vi "TestExampleCD.vi"() -> ()   [LabVIEW 2012]
uses:
  ExampleClassC/ExampleClassC.lvclass
  ExampleClassDEdge/ExampleClassDEdge.lvclass
  ExampleClassDInverse/ExampleClassDInverse.lvclass
  ExampleClassDMath/ExampleClassDKaleidoscope/ExampleClassDMath.lvclass
  ExampleClassDScaffold/ExampleClassDScaffold.lvclass
  <vilib>/Distrio/Murmex/Murmex/Murmex.lvclass
panel:
  in  "method":enum16{"Inverse", "Edge", "Math"}(ring)
  # "Test Example C & D"
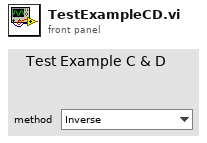
[diagram p1: front panel]
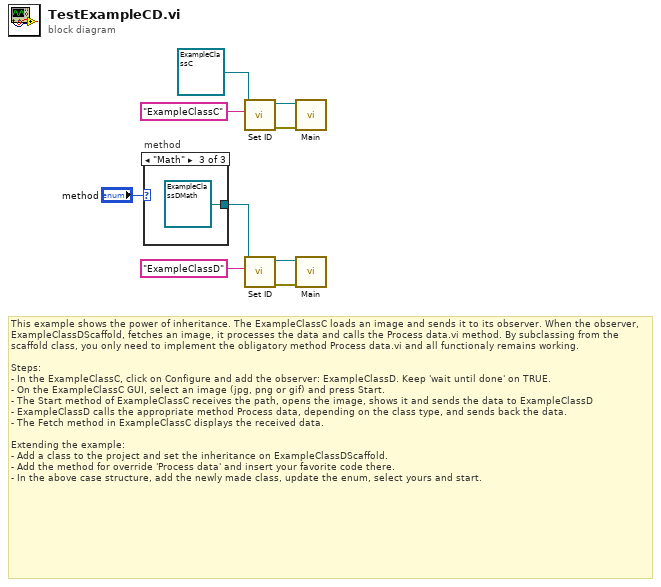
[diagram p0: block diagram]
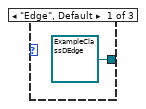
[diagram p2: hidden frame]
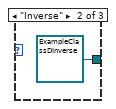
[diagram p3: hidden frame]
diagram:
  # "This example shows the power of inheritance. The ExampleClassC loads an image and sends it to its observer. When the observer, ExampleClassDScaffold, fetches an image, it processes the data and calls the Process data.vi method. By subclassing from the scaffold class, you only need to implement the obligatory method Process data.vi and all functionaly remains working.\n\nSteps:\n- In the ExampleClassC, click on Configure and add the observer: ExampleClassD. Keep 'wait until done' on TRUE.\n- On the ExampleClassC GUI, select an image (jpg, png or gif) and press Start.\n- The Start method of ExampleClassC receives the path, opens the image, shows it and sends the data to ExampleClassD\n- ExampleClassD calls the appropriate method Process data, depending on the class type, and sends back the data.\n- The Fetch method in ExampleClassC displays the received data.\n\nExtending the example:\n- Add a class to the project and set the inheritance on ExampleClassDScaffold.\n- Add the method for override 'Process data' and insert your favorite code there.\n- In the above case structure, add the newly made class, update the enum, select yours and start."
  n1 = case "method" shown="\"Math\"" "method" {
    tunnel: [refnum<class "ExampleClassDEdge.lvclass"> refnum ("ExampleClassDEdge") refnum<class "ExampleClassDInverse.lvclass"> refnum ("ExampleClassB.lvclass") refnum<class "ExampleClassDMath.lvclass"> refnum ("ExampleClassDKaleidoscope.lvclass")] -> w5
    frame "Edge", Default {
    }
    frame "Inverse" {
    }
    frame "Math" {
    }
  }
  n2 = call <vilib>:"Set ID.vi"("id"="ExampleClassC", "Murmex in"=refnum<class "ExampleClassC.lvclass"> refnum ("ExampleClassA.lvclass")) -> ("error out"=w1:errorcluster, "Murmex out"=w2:refnum<class "ExampleClassC.lvclass">)  [unwired: 8 in]
  n3 = call <vilib>:"Set ID.vi"("id"="ExampleClassD", "Murmex in"=w5) -> ("error out"=w7:errorcluster, "Murmex out"=w6:refnum<class "ExampleClassDScaffold.lvclass">)  [unwired: 8 in]
  n4 = call-dynamic "Main.vi"("error in (no error)"=w1, "ExampleClassC in"=w2) -> ()  [unwired: 8 in, 2 out]
  n5 = call-dynamic "Main.vi"("error in (no error)"=w7, "ExampleClassDScaffold in"=w6) -> ()  [unwired: 8 in, 2 out]
